vi "Estados Feeder Global.vi"() -> ()   [LabVIEW 2015]
uses:
  TypeDefs/estadosFeeder.ctl
panel:
  in  "Enum":T1
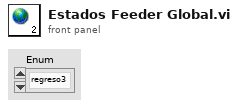
[diagram p1: front panel]
types:
  T1 = typedef "estadosFeeder.ctl" = enum16{"regreso3", "regreso2", "regreso1", "afuera2", "afuera1"}
diagram:
